vi "SetComponent.vi"(0 "reference in":refnum<class "MES_Local.lvclass">, 5 "Name":string, 7 "SN":string, 9 "BN":string, 11 "error in (no error)":errorcluster) -> (4 "reference in":refnum<class "MES_Local.lvclass">, 15 "error out":errorcluster)   [LabVIEW 2022 SP3, in "MES_Local.lvlib" / "MES_Local.lvclass"]
uses:
  MES_Local.lvclass
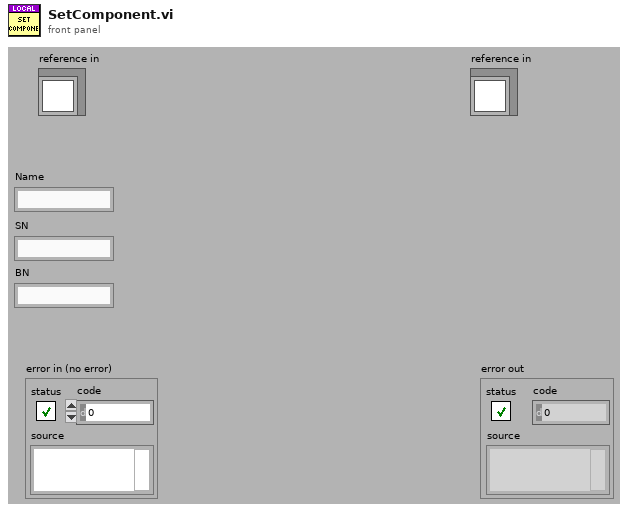
[diagram p1: front panel]
types:
  T1 = typedef "MES_Local.lvlib/MES_Local.lvclass/ObjectAttributes.ctl" = cluster{"Config":T2, "Logged_In?":bool, "AttributeNames":string[], "AttributeWritten":bool[], "ComponentNames":string[], "TestIndex":i32, "TestTag":string[], "Time Stamp":timestamp, "Employee":string, "Resource_Key":string, "Local Spec":path, "Login":refnum<class "Login_Base.lvclass">, "ReportPath":path, "Spec":T3, "StartTime":timestamp, "Role":string}
  T2 = typedef "MES_Local.lvlib/MES_Local.lvclass/Config.ctl" = cluster{"Results_Path":path}
  T3 = typedef "MES_Base.lvlibp/MES_Base.lvclass/Spec.ctl" = cluster{"Header":cluster{"Doctype":string, "Checksum":string, "DriverKey":string, "SpecId":string, "TransactionId":string, "AccountId":string, "SpecName":string, "WorkflowStep":string, "SerialNumber":string, "BatchNumber":string, "Status":enum16{"Pending", "Pass", "Fail"}, "Comment":string, "FirstFail":string, "Employee":string, "LocalMachine":string, "ResourceKey":string, "Date":string, "Time":string, "Duration":string, "DUT Position":i32}, "Components":cluster{"SerialNumber":string, "PartNumber":string, "Revision":string, "BatchNumber":string, "Name":string, "Description":string, "Attached":bool}[], "Attributes":cluster{"Name":string, "Description":string, "DataType":enum16{"NA", "String", "Boolean", "Int", "Dbl"}, "Value":variant, "DisplayFormat":string, "ReadOnly":bool, "Required":bool}[], "Tests":cluster{"Code":string, "Name":string, "Description":string, "Group":string, "IsGroup":bool, "Tag":string, "Method":string, "Parrameter":string, "DataType":enum16{"NA", "String", "Boolean", "Int", "Dbl"}, "Value":variant, "Status":enum16{"Pending", "Pass", "Fail"}, "LimitLo":variant, "LimitHi":variant, "StringMatch":string, "BooleanMatch":bool, "DisplayFormat":string, "Units":string, "TestTime":dbl}[]}
  T4 = cluster{"SerialNumber":string, "PartNumber":string, "Revision":string, "BatchNumber":string, "Name":string, "Description":string, "Attached":bool}[]
  T5 = cluster{"SerialNumber":string, "PartNumber":string, "Revision":string, "BatchNumber":string, "Name":string, "Description":string, "Attached":bool}
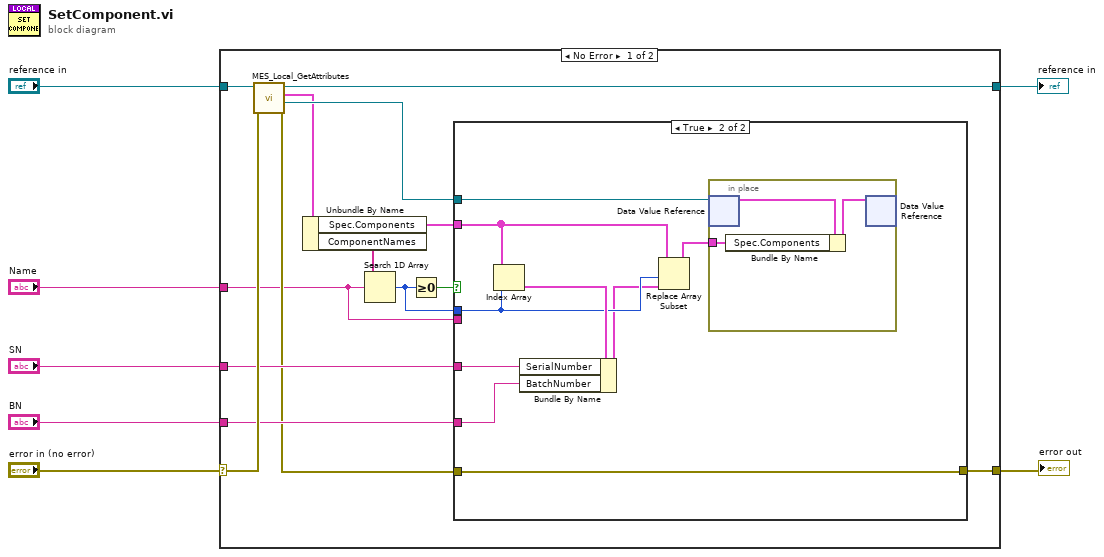
[diagram p0: block diagram]
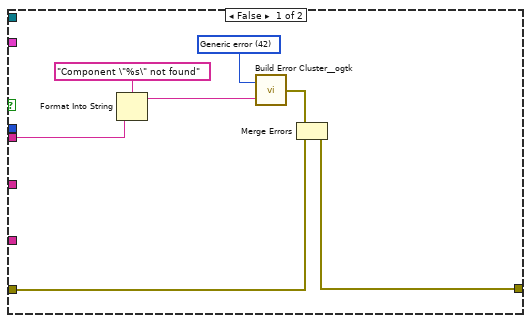
[diagram p2: hidden frame]
diagram:
  n1 = case shown="No Error" "error in (no error)" {
    selector: "error in (no error)" -> [w21 w42]
    tunnel: [w9 w42] -> w6
    tunnel: [w19 w41] -> w4
    tunnel: "reference in" -> [w20 w41]
    tunnel: "Name" -> [w8 _]
    tunnel: "SN" -> [w12 _]
    tunnel: "BN" -> [w11 _]
    frame No Error {
      n2 = call "MES_Local_GetAttributes.vi"("error in (no error)"=w21, "reference in"=w20) -> ("error out"=w10:errorcluster, "DataRef"=w14:refnum<data-value>, "Data"=w13:T1, "reference out"=w19:refnum<class "MES_Local.lvclass">)  [unwired: 6 in]
      n3 = Unbundle By Name(w13) -> ("Spec.Components"=w15:T4, "ComponentNames"=w18:string[])
      n4 = Search 1D Array(1D array=w18, element=w8) -> (index of element=w16:i32)  [unwired: 1 in]
      n5 = Greater Or Equal To 0?(x=w16) -> (x >= 0?=w17:bool)
      n6 = case shown="True" w17 {
        tunnel: w16 -> [_ w35]
        tunnel: w15 -> [_ w36]
        tunnel: w11 -> [_ w30]
        tunnel: w12 -> [_ w31]
        tunnel: w14 -> [_ w33]
        tunnel: w8 -> [w24 _]
        tunnel: [w23 w29] -> w9
        tunnel: w10 -> [w22 w29]
        frame False {
          w28 = 42 items=["No error", "Argument error", "Memory is full", "Out of zone", "End of file", "File already open", "Generic file I/O error", "File not found", "File permission error", "Disk is full", "Duplicate path", "Too many files open", "System feature not enabled", "Resource file not found", "Cannot add resource", "Resource not found", "Image not found", "Image memory error", "Pen does not exist", "Config type invalid", "Config token not found", "Config parse error", "Config memory error", "Bad external code format", "Bad external code offset", "External code not present", "Null window", "Destroy window error", "Null menu", "Print aborted", "Bad print record", "Print driver error", "Windows error during printing", "Memory error during printing", "Print dialog error", "Generic print error", "Invalid device refnum", "Device not found", "Device parameter error", "Device unit error", "Cannot open device", "Device call aborted", "Generic error", "Cancelled by user", "Object ID too low", "Object ID too high", "Object not in heap", "Unknown heap", "Unknown object (invalid DefProc)", "Unknown object (DefProc not in table)", "Message out of range", "Invalid (null) method", "Unknown message", "Manager call not supported", "Bad address", "Network operation in progress", "Network operation timed out", "Connection is busy", "Network attribute not supported", "Network error", "Address in use", "System out of memory", "Connection aborted", "Connection refused", "Not connected", "Already connected", "Connection closed", "Initialization error (interapplication manager)", "Bad occurrence", "Wait on unbound occurrence handler", "Occurrence queue overflow", "Datalog type conflict", "Unused", "Unrecognized type (interapplication manager)", "Memory corrupt", "Failed to make temporary DLL", "Old CIN version", "Drag socket not found", "Failed to load drop-object", "Failed to register OLE object", "Failed to release OLE object", "Format specifier type mismatch", "Unknown format specifier", "Too few format specifiers", "Too many format specifiers", "Scan failed", "Newer CIN version", "Error converting to variant", "Runtime menu error", "Password tampered", "Variant attribute not found", "Incompatible variant data type", "Event data is not available", "Event Store is not present", "Occurrence is not found", "Event Queue is not created", "Event info is not available", "Refnum passed is NULL", "Error retrieving Class GUID", "Error retrieving CoClass GUID", "Error retrieving TypeLib GUID.", "Bad built application magic bytes.", "Specific driver is different from the specific driver associated with the Logical Name.", "There is no session opened to the class driver.", "Max Error", "MAX - Error with config objects", "MAX - Error loading configuration", "MAX - Group not supported"]
          n7 = Format Into String(format string="Component \"%s\" not found", w24) -> (resulting string=w25:string)  [unwired: 2 in, 1 out]
          n8 = call <userlib>:"Build Error Cluster__ogtk.vi"("String to Prepend to source (\"\")"=w25, "code"=w28) -> ("error out"=w27:errorcluster)
          n9 = Merge Errors(w27, w22) -> (w23:errorcluster)
        }
        frame True {
          n10 = Index Array(array=w36, index=w35) -> (element=w37:T5)
          n11 = Bundle By Name(cluster=w37, "SerialNumber"=w31, "BatchNumber"=w30) -> (w34:T5)
          n12 = Replace Array Subset(array=w36, new element=w34, index=w35) -> (w32:T4)
          n13 = in-place {
            in-place-border: w32 -> [w38]
            n14 = in-place-dvr #1(w33) -> (w40:T1)  [unwired: 1 out]
            n15 = Bundle By Name(cluster=w40, "Spec.Components"=w38) -> (w39:T1)
            n16 = in-place-dvr #1(w39) -> ()  [unwired: 2 out]
          }
        }
      }
    }
    frame Error {
    }
  }
  "error out" <- w6
  "reference in" <- w4
